vi "getNewImagePaths.vi"(8 "error in (no error)":errorcluster, 10 "numberOfImages":i32, 11 "FileNeologist in":refnum<class "FileNeologist.lvclass">) -> (0 "error out":errorcluster, 2 "Paths":path[](array[path]), 3 "FileNeologist out":refnum<class "FileNeologist.lvclass">)   [LabVIEW 2011, in "Tools.lvlib" / "Filing.lvlib" / "FileNeologist.lvclass"]
uses:
  FileNeologist.lvclass
  FileNeologist.lvclass/FileNeologist.ctl
panel:
  out "scriptName":string
  out "imagePaths":string[](array[string])
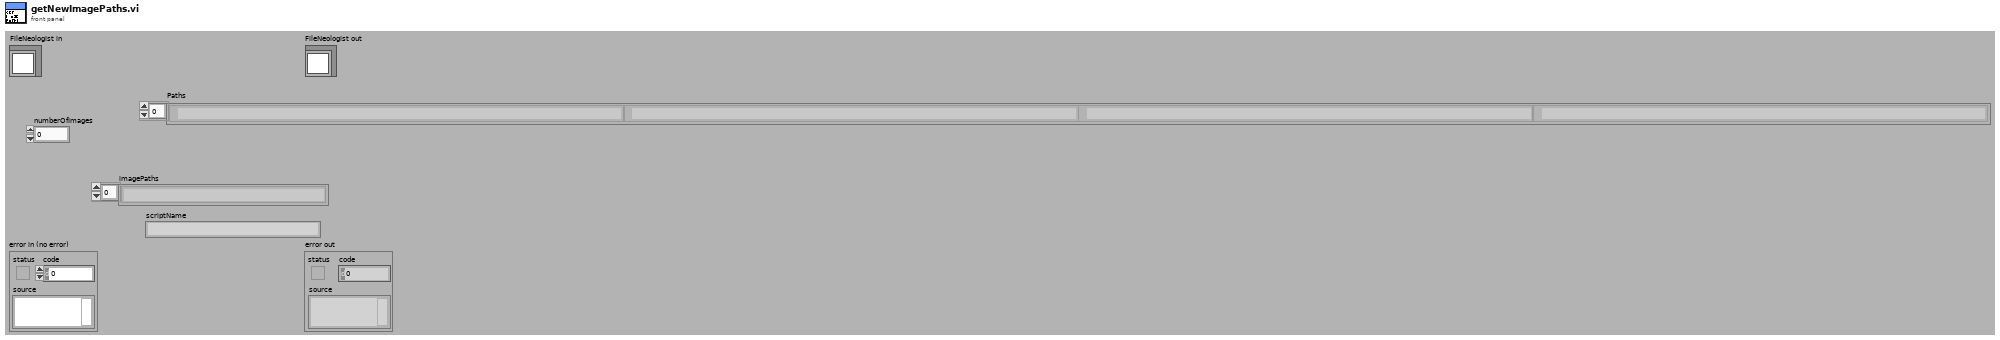
[diagram p1: front panel]
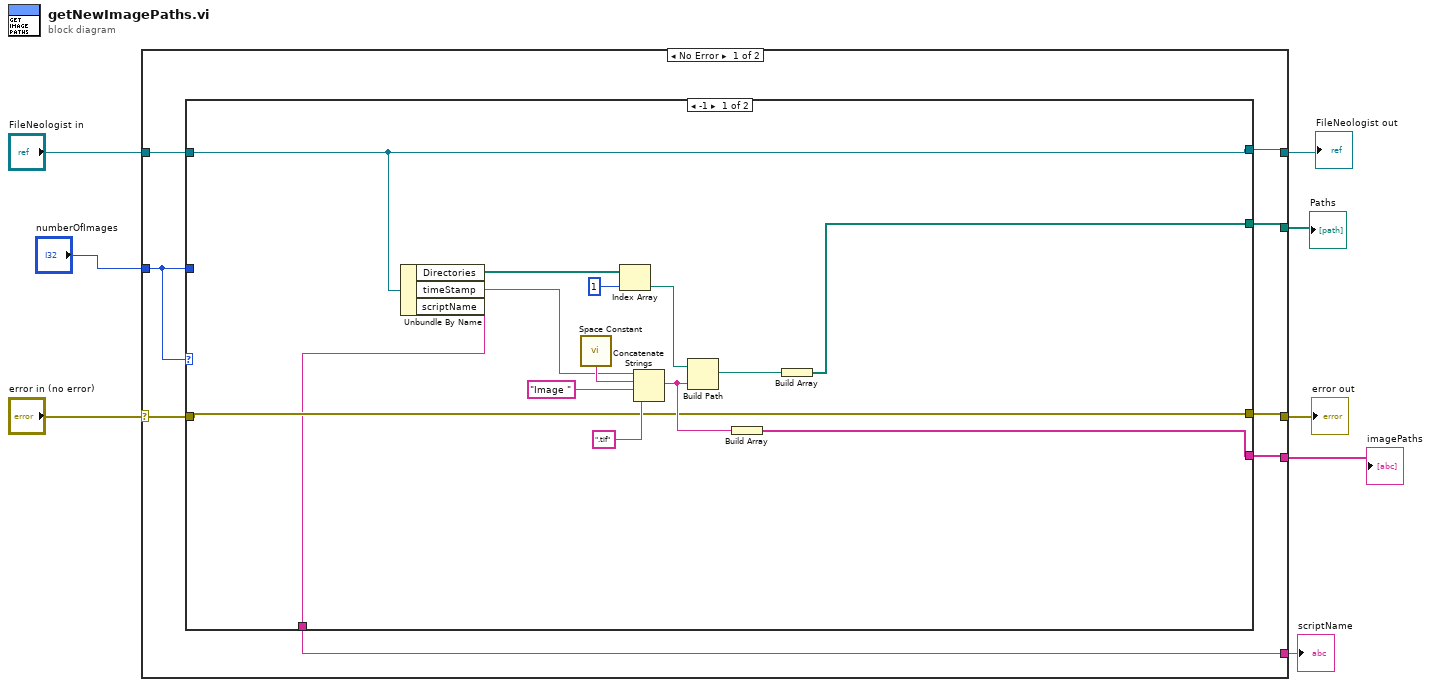
[diagram p0: block diagram]
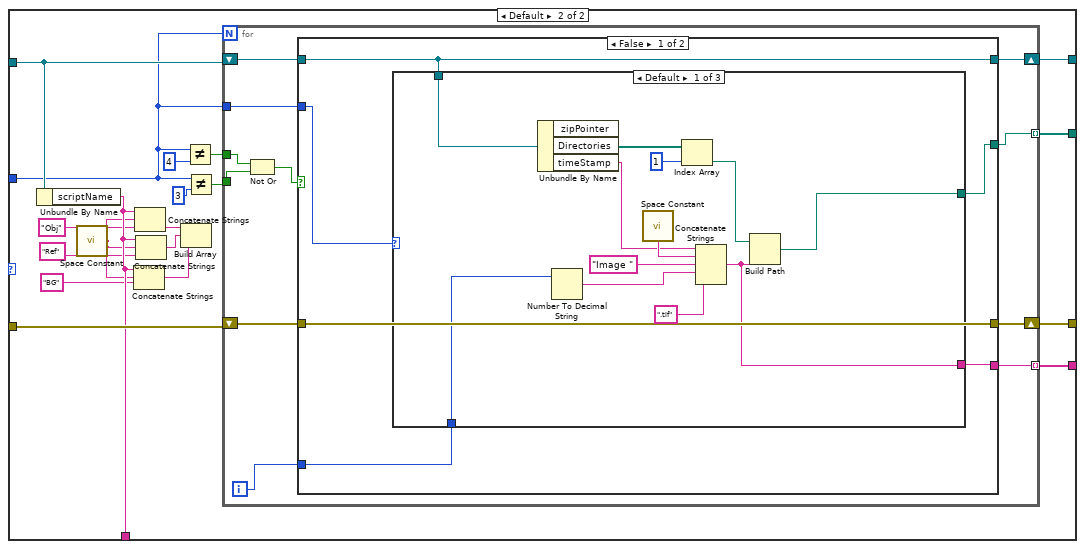
[diagram p2: hidden frame]
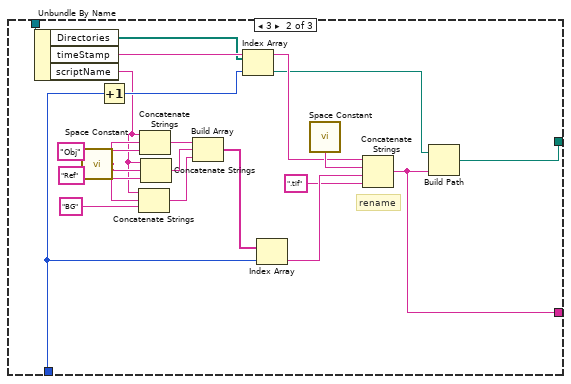
[diagram p3: hidden frame]
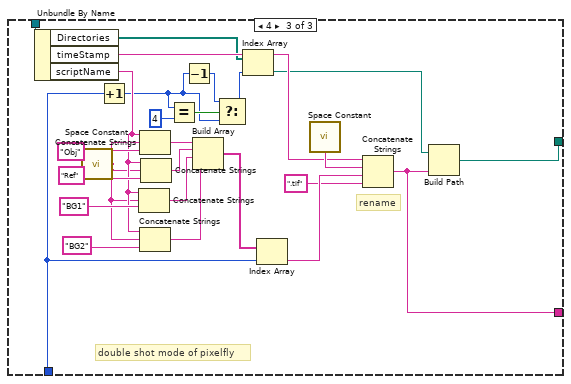
[diagram p4: hidden frame]
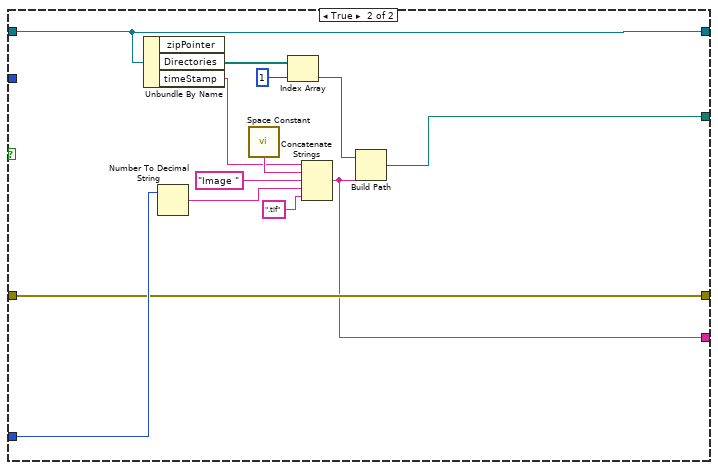
[diagram p5: hidden frame]
diagram:
  n1 = case shown="No Error" "error in (no error)" {
    selector: "error in (no error)" -> [w13 w139]
    tunnel: [w15 w139] -> w3
    tunnel: [w14 w138] -> w4
    tunnel: "FileNeologist in" -> [w12 w138]
    tunnel: [w16 _] -> w5
    tunnel: [w11 _] -> w1
    tunnel: [w10 _] -> w2
    tunnel: "numberOfImages" -> [w9 _]
    frame No Error {
      n2 = case shown="-1" w9 {
        tunnel: [w21 w49] -> w16
        tunnel: [w18 w48] -> w15
        tunnel: [w23 w47] -> w14
        tunnel: w13 -> [w18 w46]
        tunnel: w12 -> [w23 w45]
        tunnel: [w17 w44] -> w11
        tunnel: [w19 w43] -> w10
        tunnel: w9 -> [_ w31]
        frame -1 {
          n3 = Unbundle By Name(w23) -> ("Directories"=w28:path[], "timeStamp"=w29:string, "scriptName"=w17:string)
          n4 = call <vilib>:"Space Constant.vi"() -> ("String"=w30:string)
          n5 = Index Array(array=w28, index=1) -> (element=w27:path)
          n6 = Concatenate Strings(w29, w30, "Image ", ".tif") -> (w20:string)
          n7 = Build Path(base path=w27, name or relative path=w20) -> (appended path=w22:path)
          n8 = Build Array(w20) -> (w19:string[])
          n9 = Build Array(w22) -> (w21:path[])
        }
        frame Default {
          n10 = Unbundle By Name(w45) -> ("scriptName"=w44:string)
          n11 = call <vilib>:"Space Constant.vi"() -> ("String"=w36:string)
          n12 = Concatenate Strings(w44, w36, "BG") -> (w39:string)
          n13 = Concatenate Strings(w44, w36, "Obj") -> (w41:string)
          n14 = Concatenate Strings(w44, w36, "Ref") -> (w40:string)
          n15 = Build Array(w41, w40, w39) -> ()  [unwired: 1 out]
          n16 = Not Equal?(x=w31, y=4) -> (x != y?=w32:bool)
          n17 = Not Equal?(x=w31, y=3) -> (x != y?=w35:bool)
          n18 = for {
            N: w31 -> [_]
            tunnel: [w60] -> w49 mode=indexing
            shift-right: [w57] -> w47
            shift-left: w45 -> [w58]
            shift-right: [w59] -> w48
            shift-left: w46 -> [w56]
            tunnel: w35 -> [w52]
            tunnel: [w54] -> w43 mode=indexing
            tunnel: w32 -> [w53]
            tunnel: w31 -> [w50]
            i -> [w55]
            n19 = Not Or(1:w52, 2:w53) -> (0:w51:bool)
            n20 = case shown="False" w51 {
              tunnel: [w64 w128] -> w60
              tunnel: [w62 w126] -> w59
              tunnel: w58 -> [w63 w127]
              tunnel: [w63 w127] -> w57
              tunnel: w56 -> [w62 w126]
              tunnel: w55 -> [w66 w132]
              tunnel: [w65 w125] -> w54
              tunnel: w50 -> [w61 _]
              frame False {
                n21 = case shown="Default" w61 {
                  tunnel: w66 -> [w71 w94 w120]
                  tunnel: [w68 w91 w118] -> w65
                  tunnel: [w69 w89 w116] -> w64
                  tunnel: w63 -> [w72 w88 w115]
                  frame Default {
                    n22 = Unbundle By Name(w72) -> ("Directories"=w76:path[], "timeStamp"=w77:string)  [unwired: 1 out]
                    n23 = Number To Decimal String(number=w71) -> (decimal integer string=w70:string)  [unwired: 1 in]
                    n24 = call <vilib>:"Space Constant.vi"() -> ("String"=w78:string)
                    n25 = Index Array(array=w76, index=1) -> (element=w75:path)
                    n26 = Concatenate Strings(w77, w78, "Image ", w70, ".tif") -> (w68:string)
                    n27 = Build Path(base path=w75, name or relative path=w68) -> (appended path=w69:path)
                  }
                  frame 3 {
                    # "rename"
                    n28 = Unbundle By Name(w88) -> ("Directories"=w96:path[], "timeStamp"=w97:string, "scriptName"=w83:string)
                    n29 = call <vilib>:"Space Constant.vi"() -> ("String"=w84:string)
                    n30 = Increment(x=w94) -> (x+1=w93:i32)
                    n31 = Concatenate Strings(w83, w84, "BG") -> (w81:string)
                    n32 = Concatenate Strings(w83, w84, "Obj") -> (w82:string)
                    n33 = Concatenate Strings(w83, w84, "Ref") -> (w80:string)
                    n34 = Build Array(w82, w80, w81) -> (w79:string[])
                    n35 = Index Array(array=w96, index=w93) -> (element=w95:path)
                    n36 = Index Array(array=w79, index=w94) -> (element=w92:string)
                    n37 = call <vilib>:"Space Constant.vi"() -> ("String"=w98:string)
                    n38 = Concatenate Strings(w97, w98, w92, ".tif") -> (w91:string)
                    n39 = Build Path(base path=w95, name or relative path=w91) -> (appended path=w89:path)
                  }
                  frame 4 {
                    # "double shot mode of pixelfly"
                    # "rename"
                    n40 = Unbundle By Name(w115) -> ("Directories"=w122:path[], "timeStamp"=w123:string, "scriptName"=w107:string)
                    n41 = call <vilib>:"Space Constant.vi"() -> ("String"=w106:string)
                    n42 = Increment(x=w120) -> (x+1=w100:i32)
                    n43 = Concatenate Strings(w107, w106, "BG1") -> (w110:string)
                    n44 = Concatenate Strings(w107, w106, "Obj") -> (w111:string)
                    n45 = Concatenate Strings(w107, w106, "BG2") -> (w104:string)
                    n46 = Concatenate Strings(w107, w106, "Ref") -> (w109:string)
                    n47 = Equal?(x=w100, y=4) -> (x = y?=w102:bool)
                    n48 = Decrement(x=w100) -> (x-1=w101:i32)
                    n49 = Build Array(w111, w109, w110, w104) -> (w108:string[])
                    n50 = Select(t=w101, s=w102, f=w100) -> (s? t:f=w99:i32)
                    n51 = Index Array(array=w122, index=w99) -> (element=w121:path)
                    n52 = Index Array(array=w108, index=w120) -> (element=w119:string)
                    n53 = call <vilib>:"Space Constant.vi"() -> ("String"=w124:string)
                    n54 = Concatenate Strings(w123, w124, w119, ".tif") -> (w118:string)
                    n55 = Build Path(base path=w121, name or relative path=w118) -> (appended path=w116:path)
                  }
                }
              }
              frame True {
                n56 = Unbundle By Name(w127) -> ("Directories"=w135:path[], "timeStamp"=w136:string)  [unwired: 1 out]
                n57 = Number To Decimal String(number=w132) -> (decimal integer string=w130:string)  [unwired: 1 in]
                n58 = call <vilib>:"Space Constant.vi"() -> ("String"=w137:string)
                n59 = Index Array(array=w135, index=1) -> (element=w134:path)
                n60 = Concatenate Strings(w136, w137, "Image ", w130, ".tif") -> (w125:string)
                n61 = Build Path(base path=w134, name or relative path=w125) -> (appended path=w128:path)
              }
            }
          }
        }
      }
    }
    frame Error {
    }
  }
  "error out" <- w3
  "FileNeologist out" <- w4
  "Paths" <- w5
  "imagePaths" <- w2
  "scriptName" <- w1
